vi "ASI Get Exp Status.vi"(10 "pExpStatus":u32(ring) items=["ASI_EXP_IDLE", "ASI_EXP_WORKING", "ASI_EXP_SUCCESS", "ASI_EXP_FAILED"], 11 "iCameraID":i32) -> (2 "pExpStatus out":u32(ring) items=["ASI_EXP_IDLE", "ASI_EXP_WORKING", "ASI_EXP_SUCCESS", "ASI_EXP_FAILED"], 3 "function return":i32)   [LabVIEW 2012, in "ASICamera2_no_err.lvlib"]
doc: "ASICAMERA_API ASI_ERROR_CODE ASIGetExpStatus(int iCameraID, ASI_EXPOSURE_STATUS *pExpStatus);"
uses:
  <userlib>/ASICamera2_no_err/ASICamera2_no_err.lvlib
  ASICamera2.dll
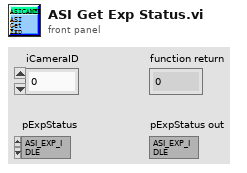
[diagram p1: front panel]
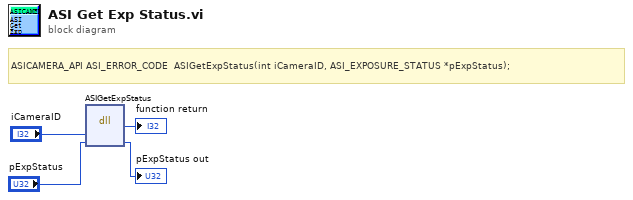
[diagram p0: block diagram]
diagram:
  # "ASICAMERA_API ASI_ERROR_CODE  ASIGetExpStatus(int iCameraID, ASI_EXPOSURE_STATUS *pExpStatus);"
  n1 = dll-call lib="ASICamera2.*" fn="ASIGetExpStatus"("iCameraID"="iCameraID", "pExpStatus"="pExpStatus") -> (→"function return":i32, "pExpStatus"=→"pExpStatus out":u32)  [unwired: 4 in, 2 out]
